vi "1D784_to_2D28_28_Int_sub.vi"(1 "1D(784)":i32[](array[numeric])) -> (0 "2D(28_28)":i32[][](array[numeric]))   [LabVIEW 2021]
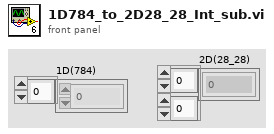
[diagram p1: front panel]
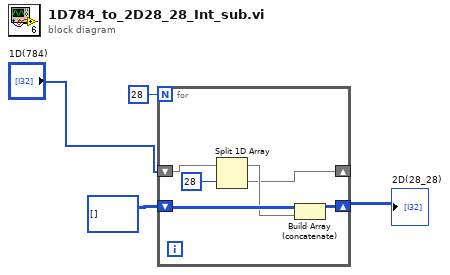
[diagram p0: block diagram]
diagram:
  n1 = for {
    N: 28 -> [_]
    shift-right: [w9] -> w1
    shift-left: i32[][] [] -> [w8]
    shift-right: [w6] -> _
    shift-left: "1D(784)" -> [w5]
    n2 = Split 1D Array(array=w5, index=28) -> (first subarray=w7:i32[], second subarray=w6:i32[])
    n3 = Build Array (concatenate)(w8, w7) -> (w9:i32[][])
  }
  "2D(28_28)" <- w1
